vi "myDyno PID.vi"(0 "Setpoint":dbl(slide) step=1.18471116e-315 scale=0.0..100.0, 2 "DC Offset":dbl min=0.0, 5 "Process Variable":dbl(slide) scale=0.0..100.0, 7 "Kp":dbl, 9 "Ki":dbl, 11 "Kd":dbl, 13 "Integral Enabled":bool=TRUE) -> (4 "Control Signal (% Duty)":dbl(slide) scale=0.0..100.0, 15 "Control Error (rps)":dbl(slide) step=1.3049304646852171e+180 scale=-40.0..40.0)   [LabVIEW 2009]
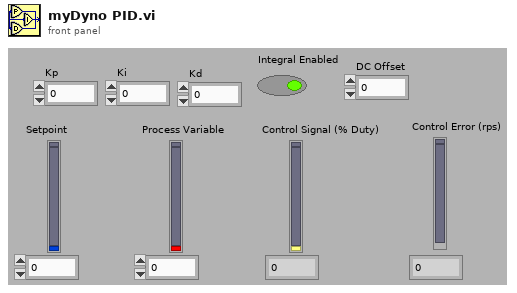
[diagram p1: front panel]
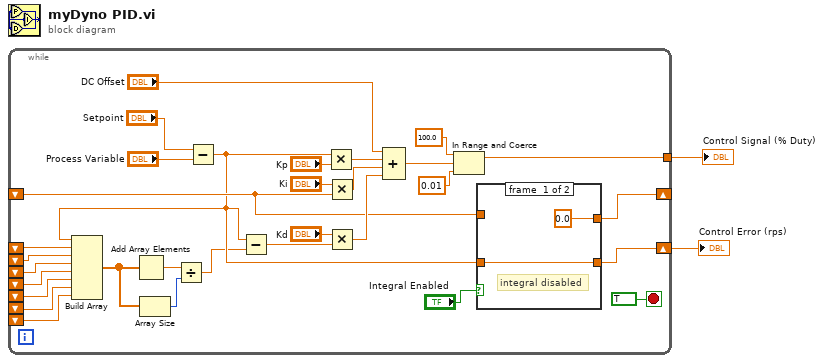
[diagram p0: block diagram]
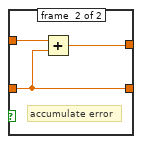
[diagram p2: hidden frame]
diagram:
  n1 = while {
    shift-right: [w18] -> _
    shift-left: _ -> [w17]
    shift-right: [w16] -> w2
    shift-left: _ -> [w15]
    shift-left: _ -> [w14]
    shift-left: _ -> [w13]
    shift-left: _ -> [w12]
    shift-left: _ -> [w11]
    shift-left: _ -> [w10]
    shift-left: _ -> [w9]
    tunnel: [w3] -> w1
    stop <- TRUE stop-if-true
    n2 = Subtract(x="Setpoint", y="Process Variable") -> (x-y=w8:dbl)
    n3 = Build Array(w8, w15, w14, w13, w12, w11, w10, w9) -> (w6:dbl[])
    n4 = Add Array Elements(numeric array=w6) -> (sum=w7:dbl)
    n5 = Array Size(array=w6) -> (size(s)=w5:i32)
    n6 = Divide(x=w7, y=w5) -> (x/y=w4:dbl)
    n7 = Subtract(x=w8, y=w4) -> (x-y=w29:dbl)
    n8 = Multiply(x=w8, y="Kp") -> (x*y=w25:dbl)
    n9 = Multiply(x="Ki", y=w17) -> (x*y=w24:dbl)
    n10 = Multiply(x="Kd", y=w29) -> (x*y=w23:dbl)
    n11 = Compound Arithmetic op=ADD("DC Offset", w25, w24, w23) -> (w28:dbl)
    n12 = In Range and Coerce(upper limit=100.0, x=w28, lower limit=0.01) -> (coerced(x)=w3:dbl)  [unwired: 1 out]
    n13 = case shown="False" "Integral Enabled" {
      tunnel: w8 -> [w34 w36]
      tunnel: [0.0 w37] -> w18
      tunnel: w17 -> [_ w38]
      tunnel: [w34 w36] -> w16
      frame #0 {
        # "integral disabled"
      }
      frame #1 {
        # "accumulate error"
        n14 = Add(x=w38, y=w36) -> (x+y=w37:dbl)
      }
    }
  }
  "Control Error (rps)" <- w2
  "Control Signal (% Duty)" <- w1
